vi "Bit Mask to Permissions.vi"(1 "Bit Mask":u32) -> (0 "Permissions":T1)   [LabVIEW 2018, in "Toolkit.lvlib"]
uses:
  Toolkit.lvlib
  Type Definitions/Permissions.ctl
  Type Definitions/Modes.ctl
  Type Definitions/Bit Mask Modes.ctl
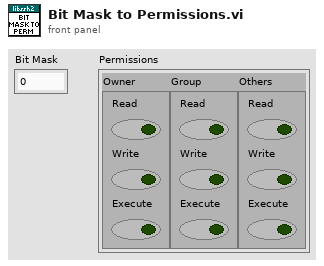
[diagram p1: front panel]
types:
  T1 = typedef "Toolkit.lvlib/Permissions.ctl" = cluster{"Owner":T2, "Group":T2, "Others":T2}
  T2 = typedef "Toolkit.lvlib/Modes.ctl" = cluster{"Read":bool, "Write":bool, "Execute":bool}
  T3 = typedef "Toolkit.lvlib/Bit Mask Modes.ctl" = u32
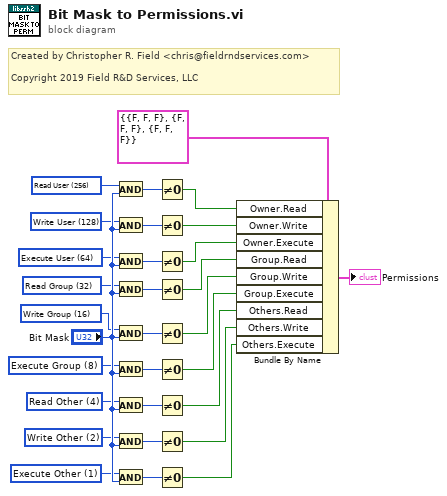
[diagram p0: block diagram]
diagram:
  w1 = T3 1 items=["Read User"=256, "Write User"=128, "Execute User"=64, "Read Group"=32, "Write Group"=16, "Execute Group"=8, "Read Other"=4, "Write Other"=2, "Execute Other"=1] ("Mode")
  w2 = T3 2 items=["Read User"=256, "Write User"=128, "Execute User"=64, "Read Group"=32, "Write Group"=16, "Execute Group"=8, "Read Other"=4, "Write Other"=2, "Execute Other"=1] ("Mode")
  w3 = T3 4 items=["Read User"=256, "Write User"=128, "Execute User"=64, "Read Group"=32, "Write Group"=16, "Execute Group"=8, "Read Other"=4, "Write Other"=2, "Execute Other"=1] ("Mode")
  w4 = T3 8 items=["Read User"=256, "Write User"=128, "Execute User"=64, "Read Group"=32, "Write Group"=16, "Execute Group"=8, "Read Other"=4, "Write Other"=2, "Execute Other"=1] ("Mode")
  w5 = T3 16 items=["Read User"=256, "Write User"=128, "Execute User"=64, "Read Group"=32, "Write Group"=16, "Execute Group"=8, "Read Other"=4, "Write Other"=2, "Execute Other"=1] ("Mode")
  w6 = T3 32 items=["Read User"=256, "Write User"=128, "Execute User"=64, "Read Group"=32, "Write Group"=16, "Execute Group"=8, "Read Other"=4, "Write Other"=2, "Execute Other"=1] ("Mode")
  w7 = T3 64 items=["Read User"=256, "Write User"=128, "Execute User"=64, "Read Group"=32, "Write Group"=16, "Execute Group"=8, "Read Other"=4, "Write Other"=2, "Execute Other"=1] ("Mode")
  w8 = T3 128 items=["Read User"=256, "Write User"=128, "Execute User"=64, "Read Group"=32, "Write Group"=16, "Execute Group"=8, "Read Other"=4, "Write Other"=2, "Execute Other"=1] ("Mode")
  w9 = T3 256 items=["Read User"=256, "Write User"=128, "Execute User"=64, "Read Group"=32, "Write Group"=16, "Execute Group"=8, "Read Other"=4, "Write Other"=2, "Execute Other"=1] ("Mode")
  # "Created by Christopher R. Field <chris@fieldrndservices.com>\n\nCopyright 2019 Field R&D Services, LLC"
  n1 = And(x=w9, y="Bit Mask") -> (x .and. y?=w28:T3)
  n2 = And(x=w8, y="Bit Mask") -> (x .and. y?=w26:T3)
  n3 = And(x=w7, y="Bit Mask") -> (x .and. y?=w22:T3)
  n4 = And(x=w6, y="Bit Mask") -> (x .and. y?=w23:T3)
  n5 = And(x=w5, y="Bit Mask") -> (x .and. y?=w24:T3)
  n6 = And(x=w4, y="Bit Mask") -> (x .and. y?=w25:T3)
  n7 = And(x=w3, y="Bit Mask") -> (x .and. y?=w15:T3)
  n8 = And(x=w2, y="Bit Mask") -> (x .and. y?=w14:T3)
  n9 = And(x=w1, y="Bit Mask") -> (x .and. y?=w13:T3)
  n10 = Not Equal To 0?(x=w28) -> (x != 0?=w27:bool)
  n11 = Not Equal To 0?(x=w26) -> (x != 0?=w21:bool)
  n12 = Not Equal To 0?(x=w22) -> (x != 0?=w20:bool)
  n13 = Not Equal To 0?(x=w23) -> (x != 0?=w19:bool)
  n14 = Not Equal To 0?(x=w24) -> (x != 0?=w18:bool)
  n15 = Not Equal To 0?(x=w25) -> (x != 0?=w17:bool)
  n16 = Not Equal To 0?(x=w15) -> (x != 0?=w12:bool)
  n17 = Not Equal To 0?(x=w14) -> (x != 0?=w11:bool)
  n18 = Not Equal To 0?(x=w13) -> (x != 0?=w10:bool)
  n19 = Bundle By Name(cluster=T1 {"Owner"={"Read"=FALSE, "Write"=FALSE, "Execute"=FALSE}, "Group"={"Read"=FALSE, "Write"=FALSE, "Execute"=FALSE}, "Others"={"Read"=FALSE, "Write"=FALSE, "Execute"=FALSE}} ("Permissions"), "Owner.Read"=w27, "Owner.Write"=w21, "Owner.Execute"=w20, "Group.Read"=w19, "Group.Write"=w18, "Group.Execute"=w17, "Others.Read"=w12, "Others.Write"=w11, "Others.Execute"=w10) -> (→"Permissions":T1)
